vi "Create IHandleGoodbye.vi"(8 "error in (no error)":errorcluster, 11 "IWampMessage":refnum<class "IWampMessage.lvclass">) -> (0 "error out":errorcluster, 3 "IHandleGoodby out":refnum<class "IHandleGoodby.lvclass">)   [LabVIEW 2020, in "wamplv.lvlib"]
uses:
  wamplv.lvlib
  SerialisedMessages/JSONMessage/WampMessage JSON.lvclass
  SerialisedMessages/MsgPackMessage/WampMessage MsgPack.lvclass
  SerialisedMessages/IWampMessage/IWampMessage.lvclass
  HandleGoodby MsgPack.lvclass
  HandleGoodby JSON/HandleGoodby JSON.lvclass
  C:/local/wamplv/Private/Requests/MessageReceivedHandlers/Goodbye/IHandleGoodby/IHandleGoodby.lvclass
  C:/local/wamplv/Private/Requests/IInternalMessage/IInternalMessage.lvclass
  C:/local/wamplv/Private/Requests/MessageReceivedHandlers/Goodbye/HandleGoodby JSON/HandleGoodby JSON.lvclass
  C:/local/wamplv/Private/Requests/MessageReceivedHandlers/IJsonMessageHandler/IJsonMessageHandler.lvclass
  C:/local/wamplv/Private/Requests/MessageReceivedHandlers/Goodbye/HandleGoodby MsgPack.lvclass
  C:/local/wamplv/Private/Requests/MessageReceivedHandlers/IMsgPackMessageHandler/IMsgPackMessageHandler.lvclass
  IHandleGoodby/IHandleGoodby.lvclass
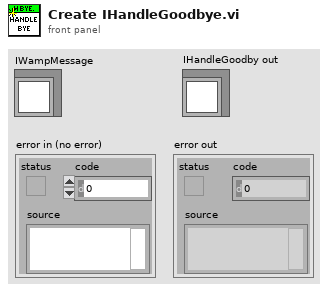
[diagram p1: front panel]
types:
  T1 = typedef "wamplv.lvlib/WAMP Client.lvclass/Serialisation.ctl" = enum16{"JSON", "MessagePack"}
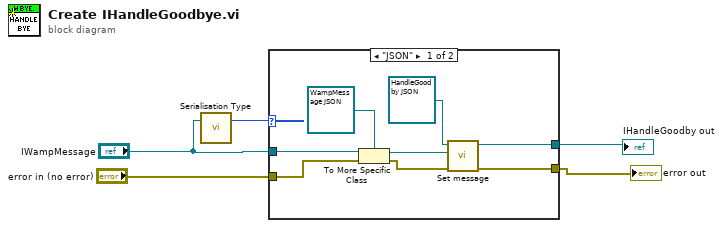
[diagram p0: block diagram]
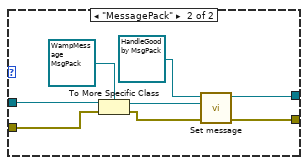
[diagram p2: hidden frame]
diagram:
  n1 = call-dynamic "Serialisation Type.vi"("IWampMessage in"="IWampMessage") -> ("Serialisation Type"=w5:T1)  [unwired: 2 in]
  n2 = case shown="\"JSON\"" w5 {
    tunnel: "IWampMessage" -> [w12 w19]
    tunnel: "error in (no error)" -> [w10 w18]
    tunnel: [w9 w16] -> w1
    tunnel: [w6 w13] -> w2
    frame "JSON" {
      n3 = To More Specific Class(target class=refnum<class "WampMessage JSON.lvclass"> refnum ("wamplv.lvlib:JSONMessage.lvclass"), reference=w12, error in=w10) -> (specific class reference=w8:refnum<class "WampMessage JSON.lvclass">, error out=w6:errorcluster)
      n4 = call-dynamic "Set message.vi"("WampMessage JSON"=w8, "IMsgPackMessageHandler in"=refnum<class "HandleGoodby JSON.lvclass"> refnum ("wamplv.lvlib:HandleGoodby JSON.lvclass")) -> ("IMsgPackMessageHandler out"=w9:refnum<class "HandleGoodby JSON.lvclass">)  [unwired: 9 in]
    }
    frame "MessagePack" {
      n5 = To More Specific Class(target class=refnum<class "WampMessage MsgPack.lvclass"> refnum ("wamplv.lvlib:MsgPackMessage.lvclass"), reference=w19, error in=w18) -> (specific class reference=w15:refnum<class "WampMessage MsgPack.lvclass">, error out=w13:errorcluster)
      n6 = call-dynamic "Set message.vi"("WampMessage MsgPack"=w15, "HandleGoodby MsgPack in"=refnum<class "HandleGoodby MsgPack.lvclass"> refnum ("wamplv.lvlib:HandleGoodby MsgPack.lvclass")) -> ("HandleGoodby MsgPack out"=w16:refnum<class "HandleGoodby MsgPack.lvclass">)  [unwired: 9 in]
    }
  }
  "error out" <- w2
  "IHandleGoodby out" <- w1
